vi "Finalize.vi"(8 "error in":errorcluster, 11 "Rx Execution Unit in":refnum<class "Rx Execution Unit.lvclass">) -> (0 "error out":errorcluster, 3 "Rx Execution Unit out":refnum<class "Rx Execution Unit.lvclass">)   [LabVIEW 2020, in "afdx_custom_device Engine.lvlib" / "Implementation.lvlib" / "Rx Execution Unit.lvclass"]
uses:
  Rx Execution Unit.lvclass
  Rx Execution Unit.lvclass/Rx Execution Unit.ctl
  AIM LabVIEW src/src/AIM664LV.lvlib
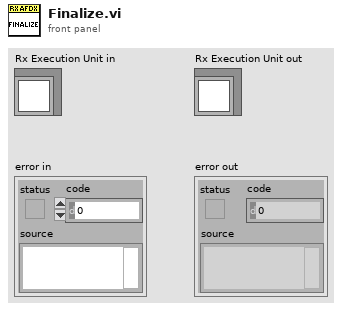
[diagram p1: front panel]
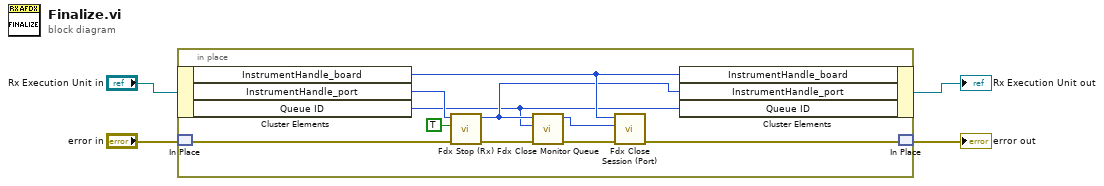
[diagram p0: block diagram]
diagram:
  n1 = in-place {
    n2 = in-place-cluster #1("Rx Execution Unit in") -> ("InstrumentHandle_board"=w10:u32, "InstrumentHandle_port"=w12:u32, "Queue ID"=w5:u32)
    n3 = in-place-match #2("error in") -> (w14:errorcluster)
    n4 = call "Fdx Stop (Rx).vi"("error in"=w14, "Force Stop?"=TRUE, "InstrumentHandle_port in"=w12) -> ("error out"=w13:errorcluster, "InstrumentHandle_port out"=w7:u32)  [unwired: 7 in]
    n5 = call "Fdx Close Monitor Queue.vi"("error in"=w13, "QueueId"=w5, "InstrumentHandle_port in"=w7) -> ("error out"=w8:errorcluster, "InstrumentHandle_port out"=w6:u32)  [unwired: 7 in]
    n6 = call "Fdx Close Session (Port).vi"("error in"=w8, "InstrumentHandle_port in"=w6, "InstrumentHandle_board in"=w10) -> ("error out"=w11:errorcluster)  [unwired: 8 in]
    n7 = in-place-cluster #1("InstrumentHandle_board"=w10, "InstrumentHandle_port"=w7, "Queue ID"=w5) -> (→"Rx Execution Unit out":refnum<class "Rx Execution Unit.lvclass">)
    n8 = in-place-match #2(w11) -> (→"error out":errorcluster)
  }
